vi "Save Data_Corrected.vi"(0 "Experiment Indicator":string, 1 "Username":string, 5 "Pixel":dbl, 7 "Scan direction":i32, 9 "Data Array":dbl[][](array[numeric]), 11 "Cell details cluster":T1={"Measure?"=TRUE, "Area (cm^2)"=0.0, "Cell Label"="", "Cell Description"="", "Cell Position"=0, "Time in rig (s)"=0.0, "Time to next scan (s)"=0.0, "Scan number"=0.0, "When did you stick it in?"=0.0, "Time between scans (s)"=0.0, "Time of the last scan (s)"=0.0, "Scan settings in queue"=0, "Sample Holder"=0.0, "User Name"=""} {"Scan settings in queue" items=["Regular", "Inverted", "MartinaSettings"]; "Time of the last scan (s)" format="%<%H:%M:%S>t"; "When did you stick it in?" format="%<%H:%M:%S>t"; "Time to next scan (s)" format="%<%H:%M:%S>t"; "Time in rig (s)" format="%<%H:%M:%S>t"}, 12 "Show me Scan \nSettings JV set":T2={"Light intensity (Suns)"=1.0, "Pre-bias time (s)"=5.0, "Maximum voltage (V)"=0.0, "Minimum voltage (V)"=-1.0, "Range Options"=0, "1st scan FB to SC?"=TRUE, "Step Size (V)"=0.01, "Source Delay (s)"=0.15, "Inverted device"=FALSE, "Measure stabilized power output"=TRUE, "Stabilzation time (s)"=60.0, "Use Vmp from JV scan"=TRUE, "Stabization voltage (V)"=0.0, "Only stabilize best pixels"=TRUE, "Number of pixels to stabilize \nper substrate"=0, "Stabilization time step (s)"=1.0, "Use max power tracking"=FALSE, "Pre-bias voltage (V)"=-1.4, "No. of data point averages"=1.0, "No. of J-V averages"=1.0, "Integration time (ms)"=200.0} {"Number of pixels to stabilize \nper substrate" items=["1", "2", "3", "4", "5", "6", "7", "8"]; "Range Options" items=["Auto Range", "Semi-Auto Range", "100 uA", "1 mA", "10 mA", "100 mA", "1A"]}, 13 "Time zero":timestamp) -> (3 "Local root path":path, 4 "Master Log":string[][](table), 6 "File path for master log":path, 8 "Server error?":bool, 10 "File path for device log":path, 14 "File path for JV data":path, 15 "File path for JV image":path)   [LabVIEW 2011]
uses:
  Typedefs/Scan settings.ctl
  Typedefs/Queue cluster.ctl
  <vilib>/Utility/file.llb/Write To Spreadsheet File (string).vi
  <vilib>/Utility/file.llb/Read From Spreadsheet File (string).vi
  <vilib>/Analysis/NI_AALPro.lvlib
panel:
  out "Vmp":dbl
  out "PCE":dbl
  out "FF":dbl
  out "Voc":dbl
  out "Jsc":dbl
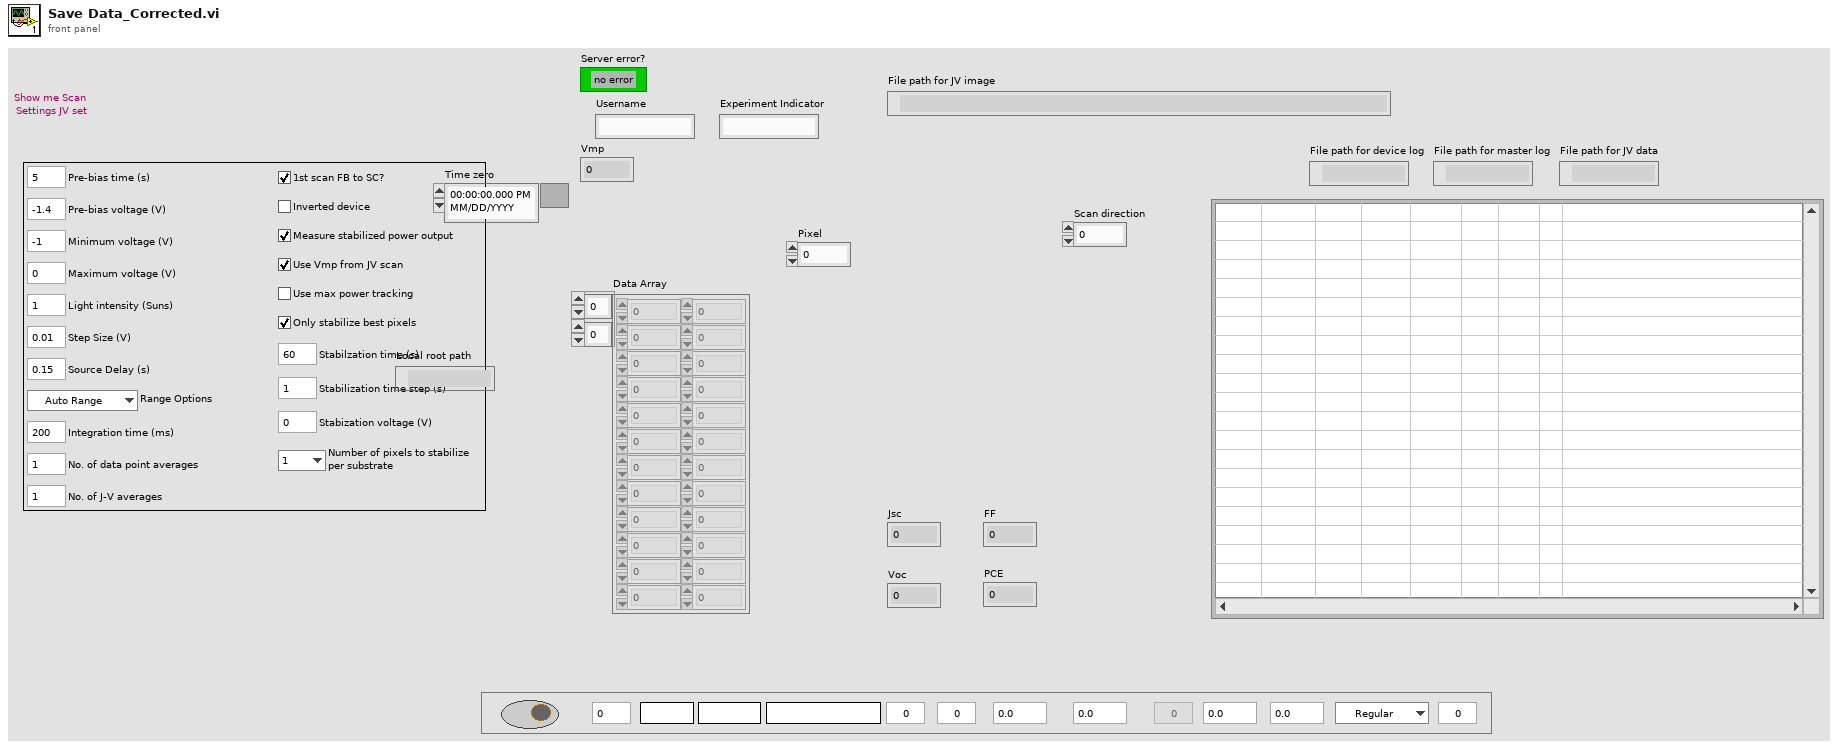
[diagram p1: front panel]
types:
  T1 = typedef "Queue cluster.ctl" = cluster{"Measure?":bool, "Area (cm^2)":dbl, "Cell Label":string, "Cell Description":string, "Cell Position":i32, "Time in rig (s)":dbl, "Time to next scan (s)":dbl, "Scan number":dbl, "When did you stick it in?":dbl, "Time between scans (s)":dbl, "Time of the last scan (s)":dbl, "Scan settings in queue":u16, "Sample Holder":dbl, "User Name":string}
  T2 = typedef "Scan settings.ctl" = cluster{"Light intensity (Suns)":dbl, "Pre-bias time (s)":dbl, "Maximum voltage (V)":dbl, "Minimum voltage (V)":dbl, "Range Options":u16, "1st scan FB to SC?":bool, "Step Size (V)":dbl, "Source Delay (s)":dbl, "Inverted device":bool, "Measure stabilized power output":bool, "Stabilzation time (s)":dbl, "Use Vmp from JV scan":bool, "Stabization voltage (V)":dbl, "Only stabilize best pixels":bool, "Number of pixels to stabilize \nper substrate":u16, "Stabilization time step (s)":dbl, "Use max power tracking":bool, "Pre-bias voltage (V)":dbl, "No. of data point averages":dbl, "No. of J-V averages":dbl, "Integration time (ms)":dbl}
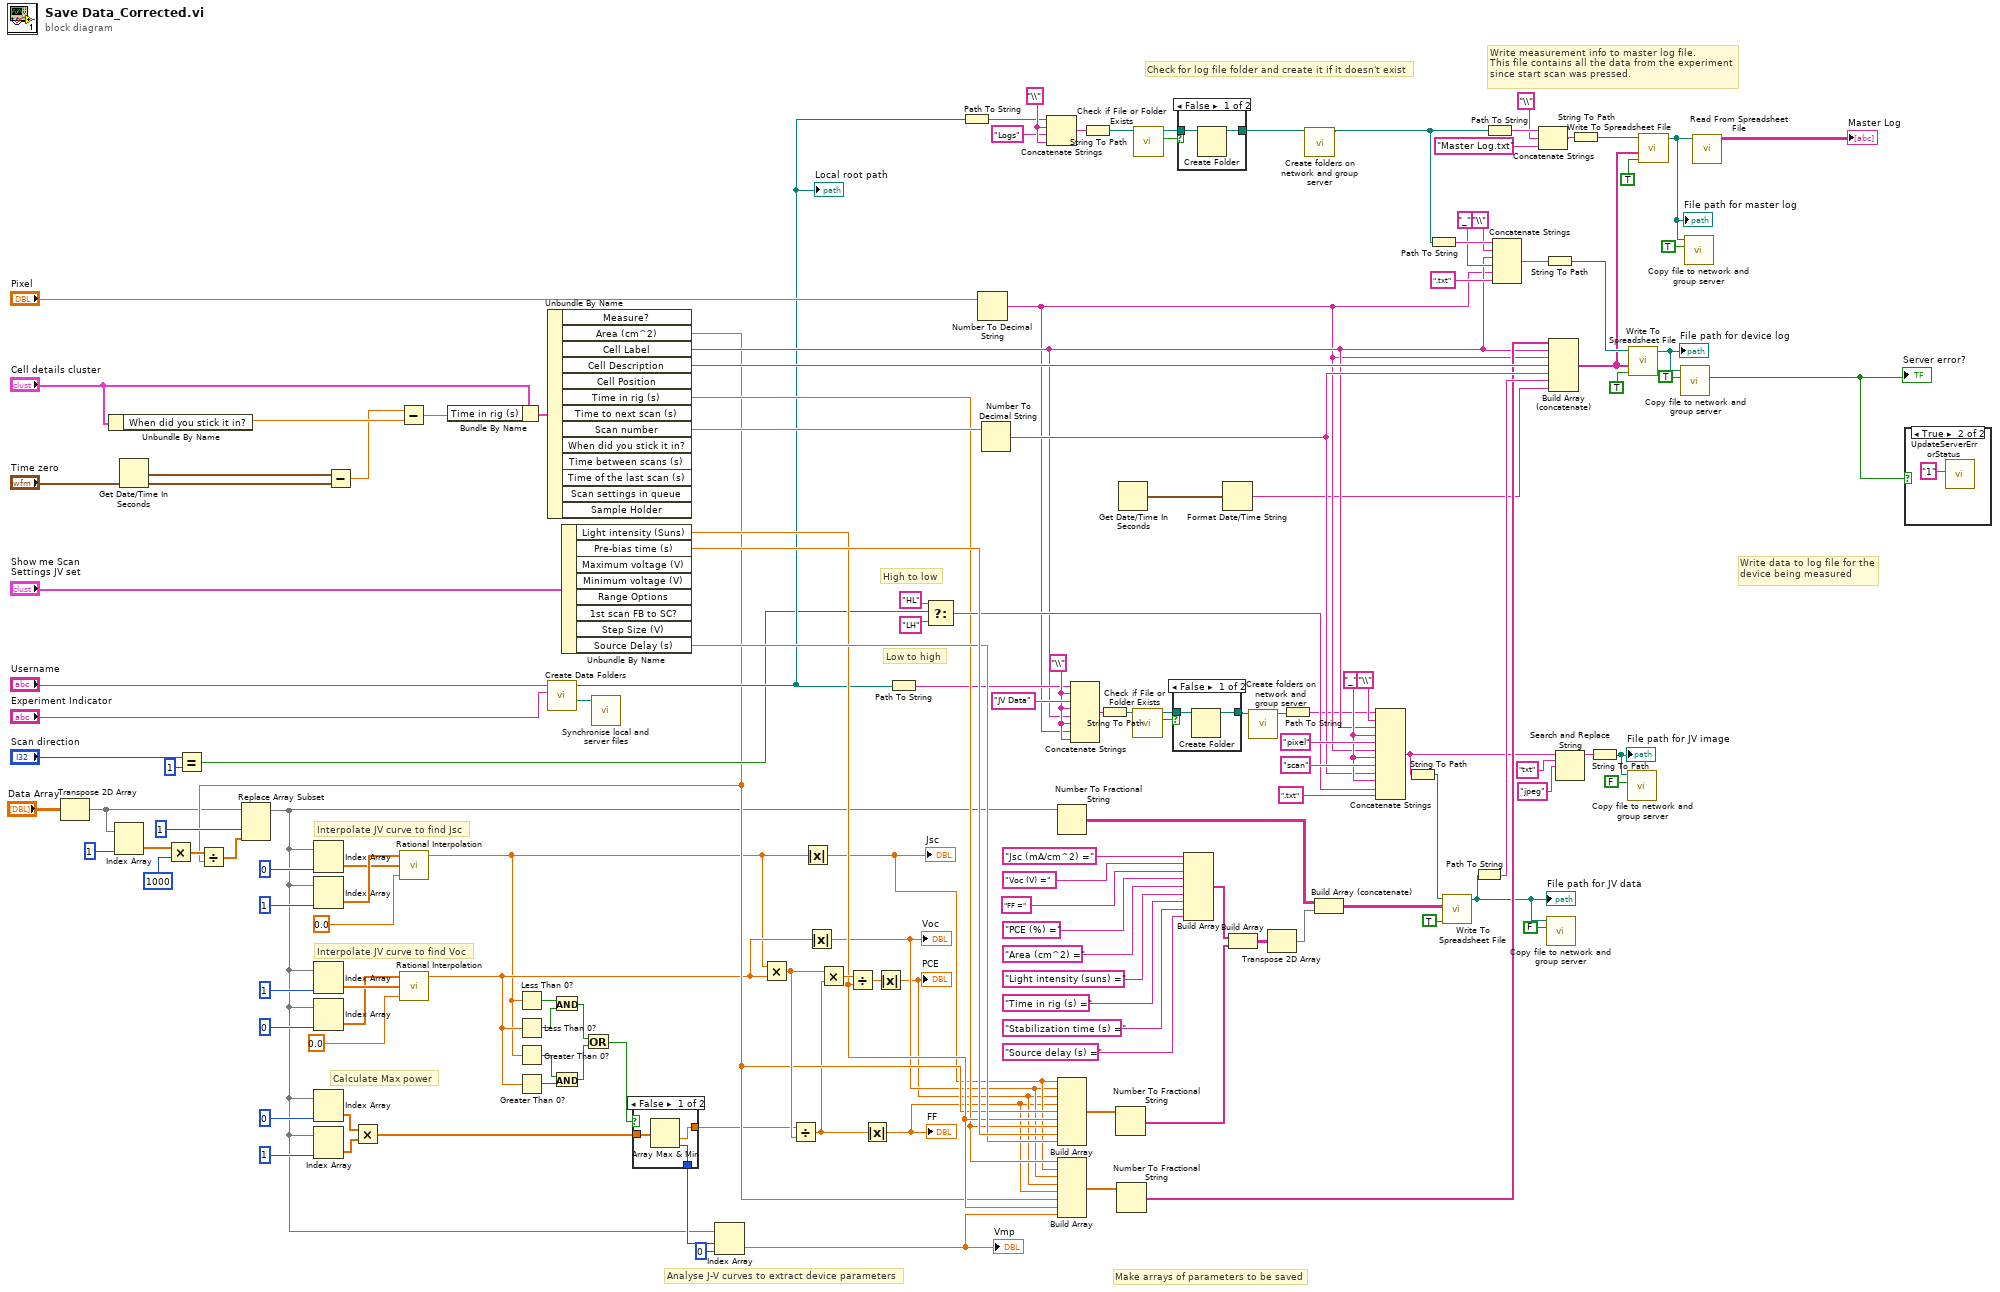
[diagram p0: block diagram]
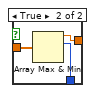
[diagram p3: hidden frame]
diagram:
  w69 = "\\"
  w95 = "\\"
  w108 = "_"
  # "Make arrays of parameters to be saved"
  # "Calculate Max power"
  # "Interpolate JV curve to find Voc"
  # "Interpolate JV curve to find Jsc"
  # "Analyse J-V curves to extract device parameters"
  # "Write data to log file for the\ndevice being measured"
  # "Write measurement info to master log file.\nThis file contains all the data from the experiment\nsince start scan was pressed."
  # "Check for log file folder and create it if it doesn't exist"
  # "Low to high"
  # "High to low"
  n1 = Transpose 2D Array(2D array="Data Array") -> (transposed array=w13:dbl[][])
  n2 = Unbundle By Name("Cell details cluster") -> ("When did you stick it in?"=w53:dbl)
  n3 = Index Array(array=w13, index (col)=1) -> (element=w35:dbl[])  [unwired: 1 in]
  n4 = Get Date/Time In Seconds() -> (seconds since 1Jan1904=w54:timestamp)
  n5 = Multiply(x=w35, y=1000) -> (x*y=w33:dbl[])
  n6 = Equal?(x="Scan direction", y=1) -> (x = y?=w44:bool)
  n7 = Subtract(x=w54, y="Time zero") -> (x-y=w52:dbl)
  n8 = Subtract(x=w52, y=w53) -> (x-y=w50:dbl)
  n9 = Bundle By Name(cluster="Cell details cluster", "Time in rig (s)"=w50) -> (w55:T1)
  n10 = Unbundle By Name(w55) -> ("Area (cm^2)"=w31:dbl, "Cell Label"=w67:string, "Cell Description"=w101:string, "Time in rig (s)"=w102:dbl, "Scan number"=w113:dbl)  [unwired: 8 out]
  n11 = Divide(x=w33, y=w31) -> (x/y=w32:dbl[])
  n12 = Replace Array Subset(array=w13, new element=w32, index (col)=1) -> (w11:dbl[][])  [unwired: 1 in]
  n13 = Index Array(array=w11, index (col)=0) -> (element=w136:dbl[])  [unwired: 1 in]
  n14 = Index Array(array=w11, index (col)=1) -> (element=w137:dbl[])  [unwired: 1 in]
  n15 = Index Array(array=w11, index (col)=1) -> (element=w135:dbl[])  [unwired: 1 in]
  n16 = Index Array(array=w11, index (col)=0) -> (element=w133:dbl[])  [unwired: 1 in]
  n17 = Index Array(array=w11, index (col)=0) -> (element=w142:dbl[])  [unwired: 1 in]
  n18 = Index Array(array=w11, index (col)=1) -> (element=w141:dbl[])  [unwired: 1 in]
  n19 = Multiply(x=w142, y=w141) -> (x*y=w134:dbl[])
  n20 = call <vilib>:"Rational Interpolation.vi"("x value"=0.0, "X"=w136, "Y"=w137) -> ("interpolation value"=w16:dbl)  [unwired: 2 out]
  n21 = call <vilib>:"Rational Interpolation.vi"("x value"=0.0, "X"=w135, "Y"=w133) -> ("interpolation value"=w17:dbl)  [unwired: 2 out]
  n22 = Less Than 0?(x=w16) -> (x < 0?=w21:bool)
  n23 = Less Than 0?(x=w17) -> (x < 0?=w18:bool)
  n24 = Greater Than 0?(x=w16) -> (x > 0?=w19:bool)
  n25 = Greater Than 0?(x=w17) -> (x > 0?=w20:bool)
  n26 = call "Create Data Folders.vi"("Experiment Indicator"="Experiment Indicator", "username"="Username") -> ("Ageing box root path"=w1:path, "Data Output Folder"=w61:path)  [unwired: 8 in]
  "Local root path" <- w61
  n27 = And(x=w21, y=w18) -> (x .and. y?=w23:bool)
  n28 = And(x=w19, y=w20) -> (x .and. y?=w22:bool)
  n29 = Unbundle By Name("Show me Scan \nSettings JV set") -> ("Light intensity (Suns)"=w103:dbl, "Pre-bias time (s)"=w118:dbl, "Source Delay (s)"=w117:dbl)  [unwired: 5 out]
  n30 = Or(x=w23, y=w22) -> (x .or. y?=w15:bool)
  n31 = call "Synchronise local and server files.vi"("Source Folder Path"=w1) -> ()  [unwired: 11 in]
  n32 = case shown="False" w15 {
    tunnel: w134 -> [w152 w155]
    tunnel: [w151 w154] -> w24
    tunnel: [w150 w153] -> w12
    frame False {
      n33 = Array Max & Min(array=w152) -> (min value=w151:dbl, min index (indices)=w150:i32)  [unwired: 2 out]
    }
    frame True {
      n34 = Array Max & Min(array=w155) -> (max value=w154:dbl, max index (indices)=w153:i32)  [unwired: 2 out]
    }
  }
  n35 = Index Array(array=w11, index (row)=w12, index (col)=0 ("disabled index (col)")) -> (element=w9:dbl)
  "Vmp" <- w9
  n36 = Multiply(x=w16, y=w17) -> (x*y=w132:dbl)
  n37 = Divide(x=w24, y=w132) -> (x/y=w25:dbl)
  n38 = Absolute Value(x=w16) -> (abs(x)=w30:dbl)
  "Jsc" <- w30
  n39 = Absolute Value(x=w17) -> (abs(x)=w29:dbl)
  "Voc" <- w29
  n40 = Multiply(x=w132, y=w25) -> (x*y=w140:dbl)
  n41 = Divide(x=w140, y=w103) -> (x/y=w28:dbl)
  n42 = Absolute Value(x=w25) -> (abs(x)=w26:dbl)
  "FF" <- w26
  n43 = Absolute Value(x=w28) -> (abs(x)=w27:dbl)
  "PCE" <- w27
  n44 = Path To String(path=w61) -> (string=w68:string)
  n45 = Select(t="HL", s=w44, f="LH") -> (s? t:f=w107:string)
  n46 = Path To String(path=w61) -> (string=w92:string)
  n47 = Number To Decimal String(number="Pixel") -> (decimal integer string=w66:string)  [unwired: 1 in]
  n48 = Number To Decimal String(number=w113) -> (decimal integer string=w100:string)  [unwired: 1 in]
  n49 = Concatenate Strings(w92, w95, "Logs", w95) -> (w93:string)
  n50 = Number To Fractional String(number=w11) -> (F-format string=w47:string[][])  [unwired: 3 in]
  n51 = Build Array(w30, w29, w27, w26, w31, w103, w102, w118, w117) -> (w127:dbl[])
  n52 = Build Array(w102, w30, w29, w27, w26, w31, w103, w9) -> (w98:dbl[])
  n53 = Concatenate Strings(w68, w69, "JV Data", w69, w67, w69, w66, w69) -> (w73:string)
  n54 = String To Path(string=w93) -> (path=w91:path)
  n55 = String To Path(string=w73) -> (path=w72:path)
  n56 = Number To Fractional String(number=w127) -> (F-format string=w125:string[])  [unwired: 3 in]
  n57 = Number To Fractional String(number=w98) -> (F-format string=w97:string[])  [unwired: 3 in]
  n58 = Get Date/Time In Seconds() -> (seconds since 1Jan1904=w8:timestamp)
  n59 = call <vilib>:"Check if File or Folder Exists.vi"("path"=w72) -> ("file or folder exists?"=w71:bool, "dup path"=w70:path)  [unwired: 8 in, 1 out]
  n60 = call <vilib>:"Check if File or Folder Exists.vi"("path"=w91) -> ("file or folder exists?"=w90:bool, "dup path"=w89:path)  [unwired: 8 in, 1 out]
  n61 = case shown="False" w71 {
    tunnel: w70 -> [w157 w158]
    tunnel: [w156 w158] -> w40
    frame False {
      n62 = Create Folder(path (use dialog)=w157) -> (created path=w156:path)  [unwired: 2 in, 2 out]
    }
    frame True {
    }
  }
  n63 = case shown="False" w90 {
    tunnel: w89 -> [w160 w161]
    tunnel: [w159 w161] -> w42
    frame False {
      n64 = Create Folder(path (use dialog)=w160) -> (created path=w159:path)  [unwired: 2 in, 2 out]
    }
    frame True {
    }
  }
  n65 = Build Array("Jsc (mA/cm^2) =", "Voc (V) =", "FF =", "PCE (%) =", "Area (cm^2) =", "Light intensity (suns) =", "Time in rig (s) =", "Stabilization time (s) =", "Source delay (s) =") -> (w126:string[])
  n66 = Format Date/Time String(seconds (now)=w8) -> (date/time string=w7:string)  [unwired: 2 in]
  n67 = Build Array(w126, w125) -> (w116:string[][])
  n68 = call "Create folders on network and group server.vi"("File path in"=w40) -> ("File path out"=w39:path)  [unwired: 10 in]
  n69 = Transpose 2D Array(2D array=w116) -> (transposed array=w115:string[][])
  n70 = Path To String(path=w39) -> (string=w65:string)
  n71 = call "Create folders on network and group server.vi"("File path in"=w42) -> ("File path out"=w41:path)  [unwired: 10 in]
  n72 = Build Array (concatenate)(w47, w115) -> (w124:string[][])
  n73 = Concatenate Strings(w65, "\\", w67, w108, "pixel", w66, w108, "scan", w100, w108, w107, ".txt") -> (w64:string)
  n74 = String To Path(string=w64) -> (path=w105:path)
  n75 = Path To String(path=w41) -> (string=w88:string)
  n76 = call-poly <vilib>:"Write To Spreadsheet File.vi"("append to file? (new file:F)"=TRUE, "2D data"=w124, "file path (dialog if empty)"=w105) -> ("new file path (Not A Path if cancelled)"=w38:path)  [unwired: 5 in]
  "File path for JV data" <- w38
  n77 = Path To String(path=w38) -> (string=w99:string)
  n78 = Path To String(path=w41) -> (string=w84:string)
  n79 = Concatenate Strings(w88, "\\", w67, "_", w66, ".txt") -> (w86:string)
  n80 = Concatenate Strings(w84, "\\", "Master Log.txt") -> (w81:string)
  n81 = String To Path(string=w86) -> (path=w85:path)
  n82 = call "Copy file to network and group server.vi"("Overwrite existing file?"=FALSE, "File path in"=w38) -> ()  [unwired: 9 in, 1 out]
  n83 = Build Array (concatenate)(w97, w67, w66, w101, w100, w99, w7) -> (w79:string[])
  n84 = Search and Replace String(input string=w64, search string="txt", replace string="jpeg") -> (result string=w63:string)  [unwired: 5 in, 3 out]
  n85 = String To Path(string=w81) -> (path=w80:path)
  n86 = String To Path(string=w63) -> (path=w58:path)
  "File path for JV image" <- w58
  n87 = call "Copy file to network and group server.vi"("Overwrite existing file?"=FALSE, "File path in"=w58) -> ()  [unwired: 9 in, 1 out]
  n88 = call-poly <vilib>:"Write To Spreadsheet File.vi"("append to file? (new file:F)"=TRUE, "1D data"=w79, "file path (dialog if empty)"=w85) -> ("new file path (Not A Path if cancelled)"=w57:path)  [unwired: 5 in]
  "File path for device log" <- w57
  n89 = call-poly <vilib>:"Write To Spreadsheet File.vi"("append to file? (new file:F)"=TRUE, "1D data"=w79, "file path (dialog if empty)"=w80) -> ("new file path (Not A Path if cancelled)"=w56:path)  [unwired: 5 in]
  "File path for master log" <- w56
  n90 = call "Copy file to network and group server.vi"("Overwrite existing file?"=TRUE, "File path in"=w57) -> ("Server error?"=w2:bool)  [unwired: 9 in]
  "Server error?" <- w2
  n91 = call "Copy file to network and group server.vi"("Overwrite existing file?"=TRUE, "File path in"=w56) -> ()  [unwired: 9 in, 1 out]
  n92 = call-poly <vilib>:"Read From Spreadsheet File.vi"("file path (dialog if empty)"=w56) -> ("all rows"=→"Master Log":string[][])  [unwired: 6 in, 4 out]
  n93 = case shown="True" w2 {
    frame False {
    }
    frame True {
      n94 = call "UpdateServerErrorStatus.vi"("Error"="1") -> ()  [unwired: 11 in]
    }
  }
